vi "NHRDCPower-bak.vi"() -> ()   [LabVIEW 2018, in "Visualization.lvlib" / "VisualizeAcPwr.lvclass"]
doc: "This VI listens for any measurement data associated with the provided PluginName and displays it to the user for analysis. The display is only suitable for data coming from the RoomAlert Plugin."
uses:
  VisualizeAcPwr.lvclass
  VisualizeBase/VisualizeBase_class/SubVIs/VisualizationOptions.ctl
  <vilib>/Utility/miscctls.llb/LVRectTypeDef.ctl
  AcPwr/AcPwrShared/clMeasurmentData.ctl
  <vilib>/event_ctls.llb/usereventprio.ctl
  VisualizeBase/VisualizeBase_class/Requests/VisUserEventType.ctl
  <extravilib>/ChannelInstances/Tag-bool/Write With Abort.vi
  <extravilib>/ChannelInstances/Tag-bool/Read With Abort.vi
  <extravilib>/ChannelInstances/Tag-bool/Instantiate.vi
  <extravilib>/ChannelInstances/Tag-bool/EndpointRead.vi
  <vilib>/Utility/error.llb/Error Cluster From Error Code.vi
  <extravilib>/ChannelInstances/Tag-bool/Endpoint.vi
  <vilib>/ErrorRing/Error Ring.xnode
  <userlib>/NIST/NISTErrorLib/NISTErrorLib.lvlib
  VisualizeBase/VisualizeBase_class/VisualizeBase.lvclass
  <extravilib>/ChannelInstances/Tag-bool.lvlib
  TestClass/Test.lvclass
  Sensor/VisualizeSensor.lvclass
  StatusAndLog/VisualizeStatus.lvclass
  AcPwr/AcPwrShared/AcPwrShared.lvlib
  AcPwr/AcPwrPlugins/ChromaPowerSupplyClass/TypeDefs/Measurements.ctl
  AcPwr/AcPwrPlugins/ChromaPowerSupplyClass/ChromaPowerSupply.lvclass
  AcPwr/AcPwrPlugins/ChromaPowerSupplyClass/TypeDefs/Device(s)Settings.ctl
  AcPwr/AcPwrModule/AcPwrModule.lvlib
  AcPwr/AcPwrPlugins/AcPwrPlugins.lvlib
panel:
  in  "Display":enum16{"Raw Data", "Voltage Vs Current"}(ring)
  in  "btnPause":bool
  out "VisualizationProperties":T1={"PauseAtStartup"=TRUE, "LogData"=FALSE, "LaunchInSubPanel"=TRUE, "FPMonitor"=0, "FPWindowBounds"={"Left"=0, "Top"=0, "Right"=0, "Bottom"=0}, "MonitorBounds"={"Left"=0, "Top"=0, "Right"=0, "Bottom"=0}, "MeasIndices"=[]}
  in  "INIFilePath":path
  in  "ModuleID":i32
  in  "Log Data":bool=TRUE
  in  "btnStop":bool
  in  "btnReset":bool
  in  "btnClearTest":bool
  in  "btnStopModule":bool
  out "XY Graph":cluster{dbl[], dbl[]}(graph)
  out "Chart":waveform(dbl)[](graph)=[{"t0"=timestamp(3657200531.6397257 s since 1904-01-01), "dt"=1.0, "Y"=[46.19]}, {"t0"=timestamp(3657200531.6397257 s since 1904-01-01), "dt"=1.0, "Y"=[2.0]}, {"t0"=timestamp(3657200531.6397257 s since 1904-01-01), "dt"=1.0, "Y"=[60.0]}]
  in  "Current":bool
  in  "Voltage":bool
  in  "Current (A)":dbl
  in  "Voltage (V)":dbl
  out "ErrorArray":errorcluster[](array[cluster])
  out "Incorrect DataType?":bool
  out "String Results":string
  in  "PluginName":string="Sensor.RoomAlert1"
  # "Set Parameter"
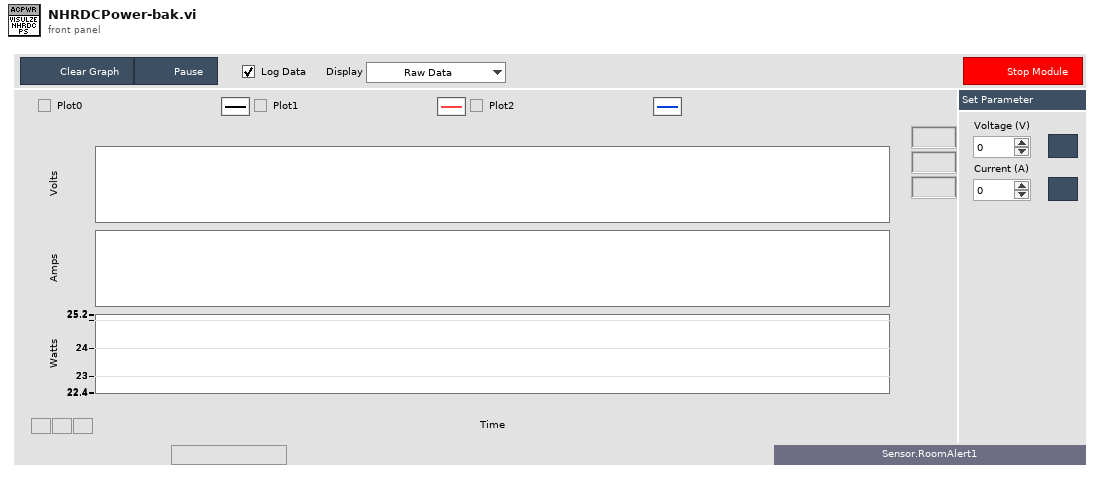
[diagram p1: front panel]
types:
  T1 = typedef "Visualization.lvlib/VisualizeBase.lvclass/VisualizationOptions.ctl" = cluster{"PauseAtStartup":bool, "LogData":bool, "LaunchInSubPanel":bool, "FPMonitor":u16, "FPWindowBounds":T2, "MonitorBounds":cluster{"Left":i16, "Top":i16, "Right":i16, "Bottom":i16}, "MeasIndices":i32[]}
  T2 = typedef "LVRectTypeDef.ctl" = cluster{"Left":i16, "Top":i16, "Right":i16, "Bottom":i16}
  T3 = enum16{"open", "open or create", "create or replace", "create", "open (read-only)"}
  T4 = typedef "Visualization.lvlib/VisualizeBase.lvclass/VisRequestEvents.ctl" = cluster{"StopRequest":refnum<user-event>, "ResetRequest":refnum<user-event>, "FP Pop In or Out":refnum<user-event>}
  T5 = typedef "AcPwrShared.lvlib/AcPwrBroadcastEvents.ctl" = cluster{"DidInit":refnum<user-event>, "StatusUpdate":refnum<user-event>, "ErrorReport":refnum<user-event>, "DidStop":refnum<user-event>, "PathToINI":refnum<user-event>, "Measurements":refnum<user-event>, "LoadConfigFile":refnum<user-event>, "GetSettings":refnum<user-event>, "SetSettings":refnum<user-event>, "GetType&ID":refnum<user-event>, "GotSettings":refnum<user-event>, "GotSettingsLV":refnum<user-event>, "ParameterSet":refnum<user-event>}
  T6 = typedef "Visualization.lvlib/VisualizeBase.lvclass/VisFrmWrkBroadcastEvents.ctl" = cluster{"StatusUpdate":refnum<user-event>, "DidStop":refnum<user-event>, "NewModuleLoaded":refnum<user-event>, "StopVisualization":refnum<user-event>}
  T7 = typedef "AcPwrShared.lvlib/clMeasurmentData.ctl" = cluster{"MeasName":string, "XML Data":string, "WaveformData":waveform(dbl)[]}
  T8 = typedef "AcPwrPlugins.lvlib/ChromaPowerSupply.lvclass/Device(s)Settings.ctl" = cluster{"Phases":cluster{"Handle":string, "Instrument Options":string, "id query (T)":bool, "reset device (T)":bool, "Timing":cluster{"TimingOn":enum16{""}, "Hours":u32, "Minutes":u32, "Seconds":dbl, "CutoffVoltage":dbl}, "Connected":bool, "Output Mode":enum16{"Voltage (DC)", "Current (DC)"}, "Voltage":dbl, "Current":dbl, "High Voltage Limit":dbl, "High Current Limit":dbl, "Power Protect":dbl, "Current Protect":dbl, "Voltage Protect":dbl, "Low Current Limit":dbl, "Low Voltage Limit":dbl, "Current Slew Rate":dbl, "Voltage Slew Rate":dbl, "Current Slew Infinite?":bool}[], "MeasName":string}
  T9 = typedef "AcPwrPlugins.lvlib/ChromaPowerSupply.lvclass/Measurements.ctl" = cluster{"Handle":string, "Name":string, "Enabled":bool, "Measurement Value":dbl, "btnMeasFetch":bool, "ProtectionStatusString":string, "Measurement Type":enum16{"Voltage", "Current", "Power"}}[]
  T10 = typedef "Visualization.lvlib/VisualizeBase.lvclass/VisUserEventType.ctl" = cluster{"BusIndex":i8, "Data":variant}
  T11 = typedef "usereventprio.ctl" = enum32{"high priority", "normal priority"}
  T12 = cluster{"Handle":string, "Instrument Options":string, "id query (T)":bool, "reset device (T)":bool, "Timing":cluster{"TimingOn":enum16{""}, "Hours":u32, "Minutes":u32, "Seconds":dbl, "CutoffVoltage":dbl}, "Connected":bool, "Output Mode":enum16{"Voltage (DC)", "Current (DC)"}, "Voltage":dbl, "Current":dbl, "High Voltage Limit":dbl, "High Current Limit":dbl, "Power Protect":dbl, "Current Protect":dbl, "Voltage Protect":dbl, "Low Current Limit":dbl, "Low Voltage Limit":dbl, "Current Slew Rate":dbl, "Voltage Slew Rate":dbl, "Current Slew Infinite?":bool}[]
  T13 = cluster{"Handle":string, "Instrument Options":string, "id query (T)":bool, "reset device (T)":bool, "Timing":cluster{"TimingOn":enum16{""}, "Hours":u32, "Minutes":u32, "Seconds":dbl, "CutoffVoltage":dbl}, "Connected":bool, "Output Mode":enum16{"Voltage (DC)", "Current (DC)"}, "Voltage":dbl, "Current":dbl, "High Voltage Limit":dbl, "High Current Limit":dbl, "Power Protect":dbl, "Current Protect":dbl, "Voltage Protect":dbl, "Low Current Limit":dbl, "Low Voltage Limit":dbl, "Current Slew Rate":dbl, "Voltage Slew Rate":dbl, "Current Slew Infinite?":bool}
  T14 = typedef "Tag-bool.lvlib/))Channel.ctl" = refnum<queue>
  T15 = typedef "sizeaction.ctl" = enum32{"Minimized", "Maximized", "Resized"}
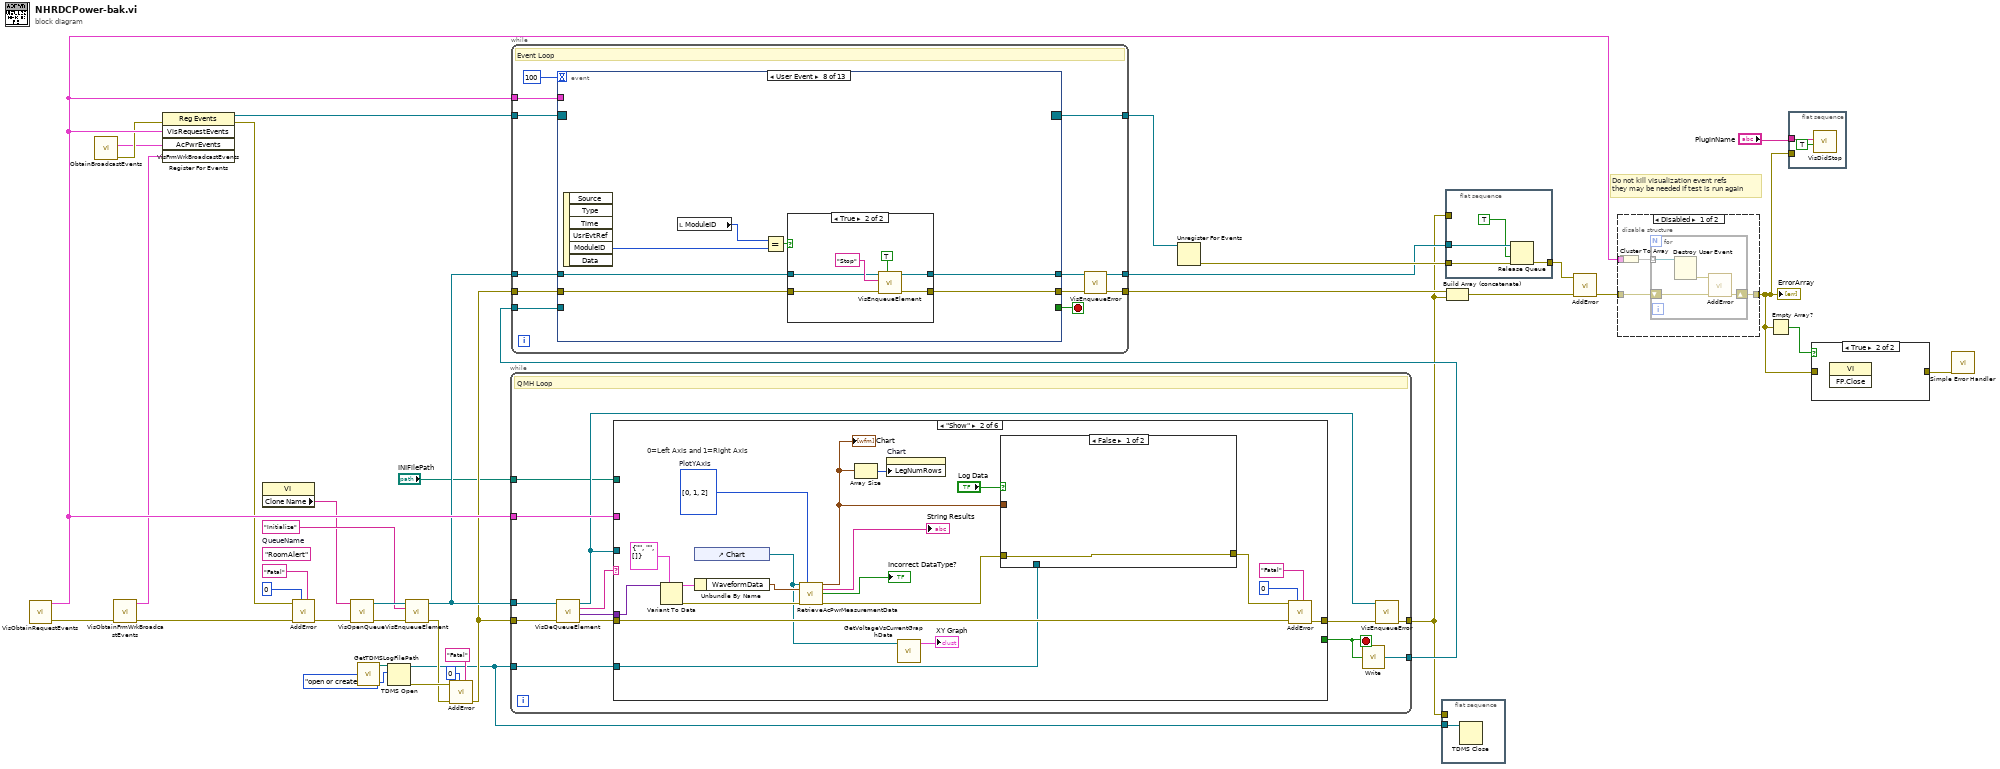
[diagram p0: block diagram]
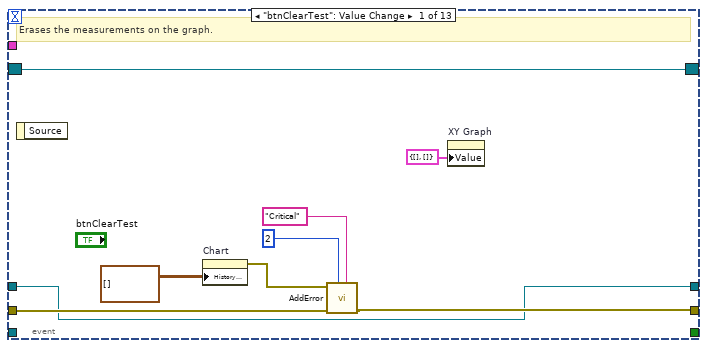
[diagram p3: hidden frame]
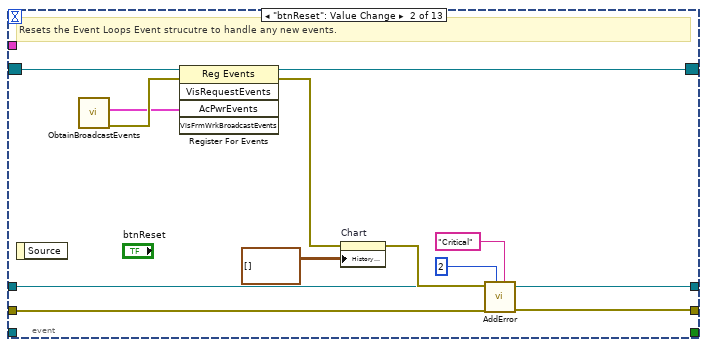
[diagram p4: hidden frame]
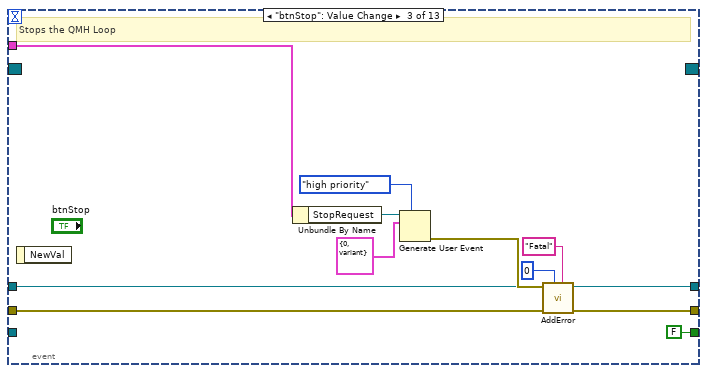
[diagram p5: hidden frame]
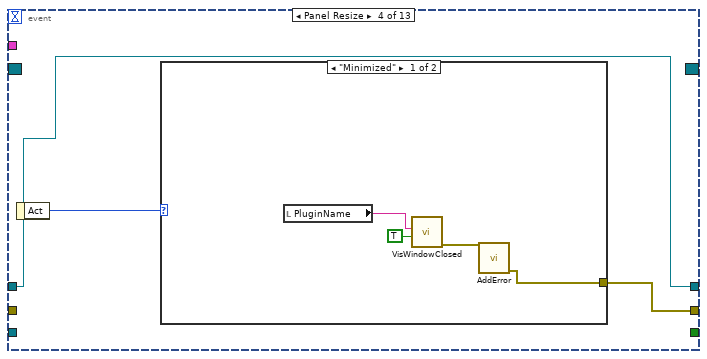
[diagram p6: hidden frame]
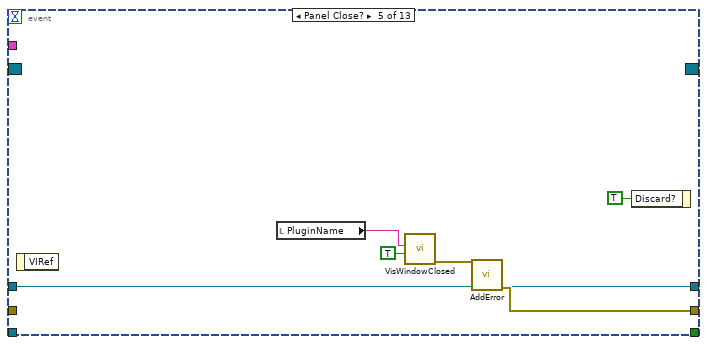
[diagram p8: hidden frame]
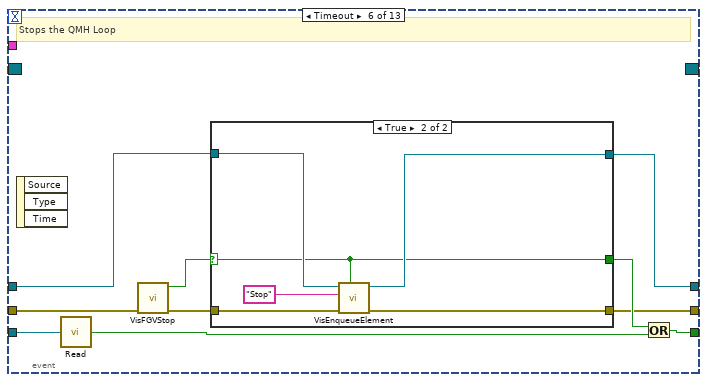
[diagram p9: hidden frame]
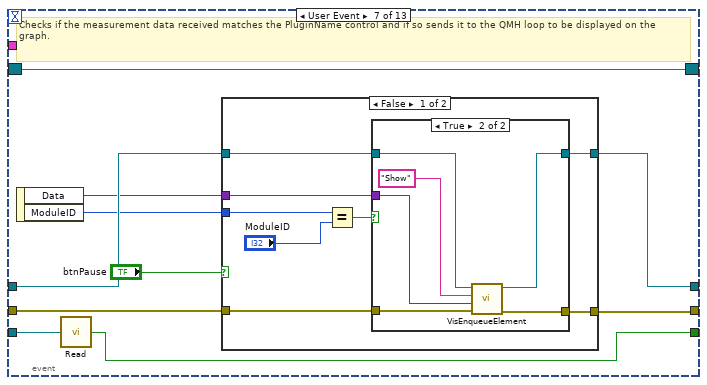
[diagram p11: hidden frame]
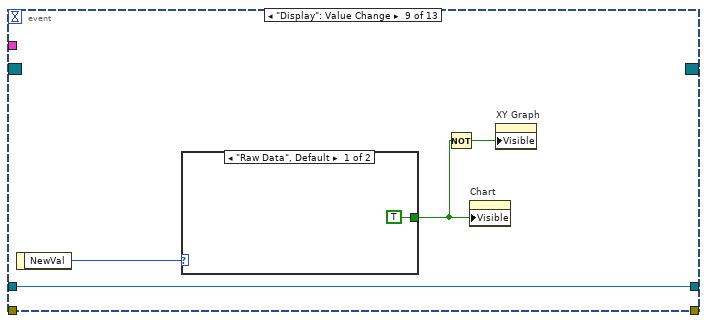
[diagram p15: hidden frame]
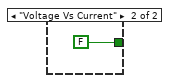
[diagram p16: hidden frame]
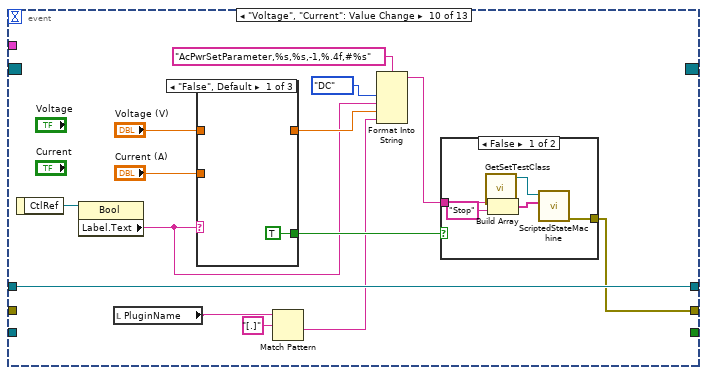
[diagram p17: hidden frame]
diagram:
  (unwired) "RoomAlert"  # QueueName
  # "Do not kill visualization event refs\nthey may be needed if test is run again"
  n1 = call "VisObtainRequestEvents.vi"() -> ("Error"=w29:errorcluster[], "VisRequestEvents"=w31:T4)  [unwired: 10 in]
  n2 = call "ObtainBroadcastEvents.vi"() -> ("error out"=w25:errorcluster, "AcPwrEvents"=w17:T5)  [unwired: 10 in]
  n3 = call "VisObtainFrmWrkBroadcastEvents.vi"("Error"=w29) -> ("Error"=w2:errorcluster[], "VisFrmWrkBroadcastEvents"=w1:T6)  [unwired: 9 in]
  n4 = register-events(error in=w25, w31, w17, w1) -> (reference out=w38:refnum<event-registration>, error out=w28:errorcluster)  [unwired: 1 in]
  n5 = property class="VI"() -> ("Clone Name"=w15:string)  [unwired: 2 in, 2 out]
  n6 = call <userlib>:"AddError.vi"("Severity"="Fatal", "Priority"=u8 0, "ErrorArray In"=w2, "error in (no error)"=w28) -> ("ErrorArray Out"=w24:errorcluster[])  [unwired: 6 in, 1 out]
  n7 = call "VisOpenQueue.vi"("Error Array In"=w24, "QueueName"=w15) -> ("Error Array Out"=w22:errorcluster[], "queue out"=w23:refnum<queue>)  [unwired: 8 in]
  n8 = call "GetTDMSLogFilePath.vi"() -> ("TDMS Log File Path"=w14:path)  [unwired: 11 in]
  n9 = TDMS Open(10:T3."open or create" ("operation (0:open)"), 11:w14) -> (0:w11:errorcluster, 3:w7:refnum<k34>)  [unwired: 5 in]
  n10 = call "VisEnqueueElement.vi"("Error Array In"=w22, "Message"="Initialize", "queue in"=w23) -> ("Error Array Out"=w10:errorcluster[], "queue out"=w20:refnum<queue>)  [unwired: 7 in]
  n11 = call <userlib>:"AddError.vi"("Severity"="Fatal", "Priority"=u8 0, "ErrorArray In"=w10, "error in (no error)"=w11) -> ("ErrorArray Out"=w9:errorcluster[])  [unwired: 6 in, 1 out]
  n12 = while {
    tunnel: w9 -> [w45]
    tunnel: [w48] -> w6
    tunnel: w20 -> [w44]
    tunnel: w31 -> [w50]
    tunnel: [w41] -> w16
    tunnel: w7 -> [w40]
    tunnel: "INIFilePath" -> [w39]
    stop <- w51 stop-if-true
    # "QMH Loop"
    n13 = call "VisDeQueueElement.vi"("Error Array In"=w45, "Queue In"=w44) -> ("Error Array Out"=w43:errorcluster[], "Data"=w46:variant, "Message"=w47:string, "Queue Out"=w42:refnum<queue>)  [unwired: 6 in]
    n14 = case shown="\"Error\"" w47 {
      selector: w47 -> [_ _ _ w122 _ _]
      tunnel: w46 -> [_ w81 w103 _ w141 _]
      tunnel: w43 -> [w62 w84 w102 w120 _ w170]
      tunnel: [w55 w85 w101 w119 w131 w169] -> w49
      tunnel: [_ _ _ _ w137 TRUE] -> w51
      tunnel: w50 -> [_ _ _ _ w136 _]
      tunnel: w42 -> [_ _ _ _ w135 _]
      tunnel: w40 -> [_ w74 _ _ _ _]
      tunnel: w39 -> [w61 _ _ _ _ w171]
      frame "Initialize" {
        n15 = property on="Chart" class="WFChart (strict)"("History Data"=waveform(dbl)[][] []) -> ()  [unwired: 2 in, 2 out]
        n16 = property on="XY Graph" class="XYGraph (strict)"("Value"=cluster{dbl[], dbl[]} {[], []} ("XY Graph")) -> ()  [unwired: 2 in, 2 out]
        n17 = call "ApplyVisOptions.vi"("INIFilePath"=w61) -> ("error out"=w65:errorcluster, "VisualizationProperties"=→"VisualizationProperties":T1)  [unwired: 9 in]
        n18 = call <userlib>:"AddError.vi"("Severity"="Inform", "ErrorArray In"=w62, "error in (no error)"=w65) -> ("ErrorArray Out"=w63:errorcluster[])  [unwired: 7 in, 1 out]
        n19 = property on="Display" class="Enum (strict)"("Val(Sgnl)"="Display") -> ()  [unwired: 2 in, 2 out]
        n20 = local read "ModuleID"() -> (w52:i32)
        n21 = call "GetSettingsRequestLV.vi"("SettingsToGet"=variant, "ModuleID"=w52) -> ("Error Out"=w54:errorcluster)  [unwired: 9 in]
        n22 = call <userlib>:"AddError.vi"("Severity"="Inform", "ErrorArray In"=w63, "error in (no error)"=w54) -> ("ErrorArray Out"=w55:errorcluster[])  [unwired: 7 in, 1 out]
      }
      frame "Show" {
        w78 = u32[] [0, 1, 2]  # PlotYAxis
        # "0=Left Axis and 1=Right Axis"
        n23 = Variant To Data(type=T7 {"MeasName"="", "XML Data"="", "WaveformData"=[]} ("MeasurmentDataCluster"), Variant=w81) -> (data=w79:T7, error out=w80:errorcluster)  [unwired: 1 in]
        n24 = control-ref of="Chart"() -> (w67:refnum<vi>)
        n25 = Unbundle By Name(w79) -> ("WaveformData"=w68:waveform(dbl)[])
        n26 = call "RetrieveAcPwrMeasurementData.vi"("WaveformChartReference"=w67, "PlotYScale"=w78, "WaveformArrayIn"=w68, "error in (no error)"=w80) -> ("WaveformArrayOut"=w70:waveform(dbl)[], "OutputString(Chroma)"=→"String Results":string, "Incorrect DataType?"=→"Incorrect DataType?":bool, "error out"=w77:errorcluster)  [unwired: 7 in, 1 out]
        "Chart" <- w70
        n27 = Array Size(array=w70) -> (size(s)=w71:i32)
        n28 = property on="Chart" class="WFChart (strict)"("LegNumRows"=w71) -> ()  [unwired: 2 in, 2 out]
        n29 = call "GetVoltageVsCurrentGraphData.vi"("WaveformChart in"=w67) -> ("Cluster"=→"XY Graph":cluster{dbl[], dbl[]})  [unwired: 9 in, 1 out]
        n30 = case shown="False" "Log Data" {
          tunnel: w77 -> [w86 w99]
          tunnel: [w86 w100] -> w76
          tunnel: w70 -> [_ w98]
          tunnel: w74 -> [_ w93]
          frame False {
          }
          frame True {
            n31 = call "PrepareWaveformDataForTDMS.vi"("error in (no error)"=w99, "WaveformArray in"=w98) -> ("error out"=w97:errorcluster, "Measurement Data"=w95:dbl[][], "Channel Names"=w96:string[], "TimeStamp"=w88:timestamp)  [unwired: 6 in]
            n32 = local read "PluginName"() -> (w91:string)
            n33 = Build Array(w88) -> (w87:timestamp[])
            n34 = TDMS Write(0:w93, 5:w91, 7:"TimeStamp" ("PluginName"), 9:w87, 11:w97) -> (4:w92:refnum<k34>, 6:w90:string, 15:w94:errorcluster)  [unwired: 1 in, 1 out]
            n35 = TDMS Write(0:w92, 5:w90, 7:w96, 9:w95, 11:w94) -> (15:w100:errorcluster)  [unwired: 1 in, 3 out]
          }
        }
        n36 = call <userlib>:"AddError.vi"("Severity"="Fatal" ("String"), "Priority"=u8 0, "ErrorArray In"=w84, "error in (no error)"=w76) -> ("ErrorArray Out"=w85:errorcluster[])  [unwired: 6 in, 1 out]
      }
      frame "GotSettings" {
        n37 = disable-structure shown="Disabled" {
          disable-tunnel: w103 -> [w111 _]
          disable-tunnel: w102 -> [w109 w115]
          disable-tunnel: [w108 w115] -> w101
          frame Disabled {
            n38 = Variant To Data(type=cluster{"Device Settings":T8, "Measurements":T9} {"Device Settings"={"Phases"=[], "MeasName"=""}, "Measurements"=[]} ("output cluster"), Variant=w111) -> (data=w112:cluster{"Device Settings":T8, "Measurements":T9}, error out=w107:errorcluster)  [unwired: 1 in]
            n39 = Unbundle By Name(w112) -> ("Device Settings.Phases"=w113:T12)
            n40 = Index Array(array=w113) -> (element=w114:T13)  [unwired: 1 in]
            n41 = Unbundle By Name(w114) -> ("Voltage"=w105:dbl, "Current"=w104:dbl)
            n42 = call <userlib>:"AddError.vi"("Severity"="Inform", "ErrorArray In"=w109, "error in (no error)"=w107) -> ("ErrorArray Out"=w108:errorcluster[])  [unwired: 7 in, 1 out]
            n43 = local write "Voltage (V)"(w105) -> ()
            n44 = local write "Current (A)"(w104) -> ()
          }
          frame Enabled {
          }
        }
      }
      frame Default {
        n45 = xnode "Error Ring"("parameter 0"=w122) -> ("error out"=w121:errorcluster)
        n46 = call <userlib>:"AddError.vi"("Severity"="Inform" ("String"), "Priority"=u8 5, "ErrorArray In"=w120, "error in (no error)"=w121) -> ("ErrorArray Out"=w119:errorcluster[], "error out"=w118:errorcluster)  [unwired: 6 in]
        n47 = call <vilib>:"Clear Errors.vi"("error in (no error)"=w118) -> ()  [unwired: 5 in, 2 out]
      }
      frame "Error" {
        n48 = Variant To Data(type=errorcluster[] [], Variant=w141) -> (data=w139:errorcluster[], error out=w130:errorcluster)  [unwired: 1 in]
        n49 = call <userlib>:"ParseErrors.vi"("ErrorArray"=w139) -> ("ErrorArray"=w138:errorcluster[])  [unwired: 8 in, 2 out]
        n50 = for {
          tunnel: w138 -> [w152] mode=indexing
          tunnel: [w146] -> w132 mode=concatenating
          tunnel: [w144] -> w137
          tunnel: w136 -> [w143]
          tunnel: w135 -> [w142]
          stop <- w144 stop-if-true
          n51 = call <userlib>:"GeneralHandler.vi"("error in (no error)"=w152) -> ("Severity"=w145:string, "Stop"=w149:bool, "Abort"=w150:bool, "Continue"=w151:bool)  [unwired: 6 in, 1 out]
          n52 = Build Array(w151, w150, w149) -> (w148:bool[])
          n53 = Boolean Array To Number(Boolean array=w148) -> (number=w147:u32)
          n54 = case shown="1" w147 {
            tunnel: [_ _ w157 w166] -> w146
            tunnel: w145 -> [_ _ _ w159]
            tunnel: [_ _ _ w161] -> w144
            tunnel: w143 -> [_ _ _ w160]
            tunnel: w142 -> [_ _ w153 _]
            frame 0, Default {
              # "No Dialog"
            }
            frame 1 {
              # "Continue"
            }
            frame 2 {
              # "Abort, Flush Queue"
              n55 = Flush Queue(queue=w153) -> (error out=w156:errorcluster)  [unwired: 1 in, 2 out]
              n56 = call <userlib>:"AddError.vi"("Severity"="Critical" ("String"), "Priority"=u8 1, "error in (no error)"=w156) -> ("ErrorArray Out"=w157:errorcluster[])  [unwired: 7 in, 1 out]
            }
            frame 4 {
              # "Stop"
              n57 = Unbundle By Name(w160) -> ("StopRequest"=w167:refnum<user-event>)
              n58 = Equal?(x=w159, y="Fatal" ("x")) -> (x = y?=w161:bool)
              n59 = Generate User Event(priority (normal)=usereventprio."high priority", user event=w167, event data cluster=T10 {"BusIndex"=0, "Data"=variant} ("event data")) -> (error out=w165:errorcluster)  [unwired: 1 in, 1 out]
              n60 = call <userlib>:"AddError.vi"("error in (no error)"=w165) -> ("ErrorArray Out"=w166:errorcluster[], "error out"=w162:errorcluster)  [unwired: 9 in]
              n61 = call <vilib>:"Clear Errors.vi"("error in (no error)"=w162) -> ()  [unwired: 5 in, 2 out]
            }
          }
        }
        n62 = call <userlib>:"AddError.vi"("Severity"="Critical", "Priority"=u8 2, "ErrorArray In"=w132, "error in (no error)"=w130) -> ("ErrorArray Out"=w131:errorcluster[])  [unwired: 6 in, 1 out]
      }
      frame "Stop" {
        n63 = local read "VisualizationProperties"() -> (w168:T1)
        n64 = call "WriteVisOptionsToINIFile.vi"("Visualization Options"=w168, "INIFilePath"=w171) -> ("error out"=w172:errorcluster)  [unwired: 8 in, 1 out]
        n65 = call <userlib>:"AddError.vi"("Severity"="Inform", "ErrorArray In"=w170, "error in (no error)"=w172) -> ("ErrorArray Out"=w169:errorcluster[])  [unwired: 7 in, 1 out]
      }
    }
    n66 = call <extravilib>:"Write.vi"("element"=w51) -> ("channel"=w41:T14)  [unwired: 1 out]
    n67 = call "VisEnqueueError.vi"("Error Array In"=w49, "Queue in"=w42) -> ("Error Array Out"=w48:errorcluster[])  [unwired: 8 in, 1 out]
  }
  n68 = while {
    tunnel: w38 -> [w186]
    tunnel: [w180] -> w36
    tunnel: [w184] -> w37
    tunnel: w31 -> [w183]
    tunnel: w9 -> [w182]
    tunnel: w20 -> [w181]
    tunnel: [w177] -> w19
    tunnel: w16 -> [w175]
    stop <- w185 stop-if-true
    # "Event Loop"
    n69 = event shown="[11] \"btnStopModule\": Value Change" {
      selector: w186 -> [w189 w207 _ _ _ _ w256 _ _ _ _ _ _]
      dyn-events: [w189 w206 _ _ _ _ w256 _ _ _ _ _ _] -> w184
      timeout: 100 -> [_ _ _ _ _ _ _ _ _ _ _ _ _]
      tunnel: [_ _ FALSE ("Priority? (F)") _ _ w232 w253 _ _ _ _ _ _] -> w185
      tunnel: [w192 w204 w211 w220 w227 w234 w258 w282 _ w300 w328 w339 w349] -> w179
      tunnel: w183 -> [_ _ w210 _ _ _ _ _ _ _ _ _ _]
      tunnel: w182 -> [w193 w205 w218 _ _ w237 w259 w281 _ _ w326 _ w348]
      tunnel: w181 -> [w187 w197 w208 w219 w226 w236 w260 w284 w294 w312 w325 w338 w351]
      tunnel: [w187 w197 w208 w219 w226 w235 w257 w283 w294 w312 w327 w338 w350] -> w178
      tunnel: w175 -> [_ _ _ _ _ w241 w254 _ _ _ _ _ _]
      event "btnClearTest": Value Change {
        # "Erases the measurements on the graph."
        n70 = event-data() -> ()  [unwired: 1 in, 1 out]
        n71 = property on="Chart" class="WFChart (strict)"("History Data"=waveform(dbl)[][] []) -> (error out=w191:errorcluster)  [unwired: 2 in, 1 out]
        n72 = call <userlib>:"AddError.vi"("Severity"="Critical", "Priority"=u8 2, "ErrorArray In"=w193, "error in (no error)"=w191) -> ("ErrorArray Out"=w192:errorcluster[])  [unwired: 6 in, 1 out]
        n73 = property on="XY Graph" class="XYGraph (strict)"("Value"=cluster{dbl[], dbl[]} {[], []} ("XY Graph")) -> ()  [unwired: 2 in, 2 out]
      }
      event "btnReset": Value Change {
        # "Resets the Event Loops Event strucutre to handle any new events."
        n74 = event-data() -> ()  [unwired: 1 in, 1 out]
        n75 = call "ObtainBroadcastEvents.vi"() -> ("error out"=w198:errorcluster, "AcPwrEvents"=w196:T5)  [unwired: 10 in]
        n76 = register-events(reference=w207, error in=w198, w196) -> (reference out=w206:refnum<event-registration>, error out=w200:errorcluster)  [unwired: 2 in]
        n77 = property on="Chart" class="WFChart (strict)"(error in=w200, "History Data"=waveform(dbl)[][] []) -> (error out=w199:errorcluster)  [unwired: 1 in, 1 out]
        n78 = call <userlib>:"AddError.vi"("Severity"="Critical", "Priority"=u8 2, "ErrorArray In"=w205, "error in (no error)"=w199) -> ("ErrorArray Out"=w204:errorcluster[])  [unwired: 6 in, 1 out]
      }
      event "btnStop": Value Change {
        # "Stops the QMH Loop"
        n79 = event-data() -> ()  [unwired: 1 in, 1 out]
        n80 = Unbundle By Name(w210) -> ("StopRequest"=w216:refnum<user-event>)
        n81 = Generate User Event(priority (normal)=usereventprio."high priority", user event=w216, event data cluster=T10 {"BusIndex"=0, "Data"=variant} ("event data")) -> (error out=w217:errorcluster)  [unwired: 1 in, 1 out]
        n82 = call <userlib>:"AddError.vi"("Severity"="Fatal" ("String"), "Priority"=u8 0, "ErrorArray In"=w218, "error in (no error)"=w217) -> ("ErrorArray Out"=w211:errorcluster[])  [unwired: 6 in, 1 out]
      }
      event Panel Resize {
        n83 = event-data() -> ("Act"=w221:T15)  [unwired: 1 in]
        n84 = case shown="\"Minimized\"" w221 {
          tunnel: [w222 _] -> w220
          frame "Minimized" {
            n85 = local read "PluginName"() -> (w224:string)
            n86 = call "VisWindowClosed.vi"("Window Closed?"=TRUE ("Window Minimized or Clozed?"), "Module Name"=w224) -> ("error out"=w225:errorcluster)  [unwired: 9 in]
            n87 = call <userlib>:"AddError.vi"("error in (no error)"=w225) -> ("ErrorArray Out"=w222:errorcluster[])  [unwired: 9 in, 1 out]
          }
          frame "Maximized", Default {
          }
        }
      }
      event Panel Close? {
        n88 = event-data() -> ()  [unwired: 1 in, 1 out]
        n89 = local read "PluginName"() -> (w228:string)
        n90 = call "VisWindowClosed.vi"("Window Closed?"=TRUE ("Window Minimized or Clozed?"), "Module Name"=w228) -> ("error out"=w229:errorcluster)  [unwired: 9 in]
        n91 = call <userlib>:"AddError.vi"("error in (no error)"=w229) -> ("ErrorArray Out"=w227:errorcluster[])  [unwired: 9 in, 1 out]
        n92 = event-data("Discard?"=TRUE) -> ()  [unwired: 1 in, 1 out]
      }
      event Timeout {
        # "Stops the QMH Loop"
        n93 = event-data() -> ()  [unwired: 1 in, 3 out]
        n94 = call <extravilib>:"Read.vi"("channel"=w241) -> ("element"=w233:bool)  [unwired: 1 in, 1 out]
        n95 = call "VisFGVStop.vi"("Error In"=w237) -> ("Error Out"=w239:errorcluster[], "Value"=w240:bool)  [unwired: 9 in]
        n96 = case shown="False" w240 {
          selector: w240 -> [w242 w245]
          tunnel: [w244 w248] -> w234
          tunnel: w239 -> [w244 w249]
          tunnel: w236 -> [w243 w247]
          tunnel: [w243 w246] -> w235
          tunnel: [w242 w245] -> w238
          frame False {
          }
          frame True {
            n97 = call "VisEnqueueElement.vi"("Priority? (F)"=w245, "Error Array In"=w249, "Message"="Stop", "queue in"=w247) -> ("Error Array Out"=w248:errorcluster[], "queue out"=w246:refnum<queue>)  [unwired: 6 in]
          }
        }
        n98 = Or(x=w238, y=w233) -> (x .or. y?=w232:bool)
      }
      event User Event {
        # "Checks if the measurement data received matches the PluginName control and if so sends it to the QMH loop to be displayed on the graph."
        n99 = event-data() -> ("Data"=w255:variant, "ModuleID"=w252:i32)  [unwired: 1 in]
        n100 = call <extravilib>:"Read.vi"("channel"=w254) -> ("element"=w253:bool)  [unwired: 1 in, 1 out]
        n101 = case shown="False" "btnPause" {
          tunnel: w260 -> [w268 w278]
          tunnel: w259 -> [w267 w277]
          tunnel: [w266 w277] -> w258
          tunnel: [w265 w278] -> w257
          tunnel: w255 -> [w264 _]
          tunnel: w252 -> [w261 _]
          frame False {
            n102 = Equal?(x=w261, y="ModuleID") -> (x = y?=w263:bool)
            n103 = case shown="True" w263 {
              tunnel: [w269 w275] -> w266
              tunnel: w268 -> [w270 w274]
              tunnel: w267 -> [w269 w276]
              tunnel: [w270 w272] -> w265
              tunnel: w264 -> [_ w273]
              frame False {
              }
              frame True {
                n104 = call "VisEnqueueElement.vi"("Error Array In"=w276, "Data"=w273, "Message"="Show", "queue in"=w274) -> ("Error Array Out"=w275:errorcluster[], "queue out"=w272:refnum<queue>)  [unwired: 6 in]
              }
            }
          }
          frame True {
          }
        }
      }
      event User Event {
        n105 = event-data() -> ("ModuleID"=w280:i32)  [unwired: 1 in, 5 out]
        n106 = local read "ModuleID"() -> (w279:i32)
        n107 = Equal?(x=w279, y=w280) -> (x = y?=w285:bool)
        n108 = case shown="True" w285 {
          tunnel: [w286 w291] -> w282
          tunnel: [w287 w290] -> w283
          tunnel: w284 -> [w287 w289]
          tunnel: w281 -> [w286 w288]
          frame False {
          }
          frame True {
            n109 = call "VisEnqueueElement.vi"("Priority? (F)"=TRUE, "Error Array In"=w288, "Message"="Stop", "queue in"=w289) -> ("Error Array Out"=w291:errorcluster[], "queue out"=w290:refnum<queue>)  [unwired: 6 in]
          }
        }
      }
      event "Display": Value Change {
        n110 = event-data() -> ("NewVal"=w297:enum16{"Raw Data", "Voltage Vs Current"})  [unwired: 1 in]
        n111 = case shown="\"Raw Data\", Default" w297 {
          tunnel: [TRUE FALSE] -> w296
          frame "Raw Data", Default {
          }
          frame "Voltage Vs Current" {
          }
        }
        n112 = Not(x=w296) -> (.not. x?=w295:bool)
        n113 = property on="Chart" class="WFChart (strict)"("Visible"=w296) -> ()  [unwired: 2 in, 2 out]
        n114 = property on="XY Graph" class="XYGraph (strict)"("Visible"=w295) -> ()  [unwired: 2 in, 2 out]
      }
      event "Voltage", "Current": Value Change {
        n115 = event-data() -> ("CtlRef"=w313:refnum<vi>)  [unwired: 1 in]
        n116 = property class="Bool"(reference=w313) -> ("Label.Text"=w302:string)  [unwired: 1 in, 2 out]
        n117 = local read "PluginName"() -> (w305:string)
        n118 = case shown="\"False\", Default" w302 {
          tunnel: "Voltage (V)" -> [_ w320 _]
          tunnel: "Current (A)" -> [_ _ w321]
          tunnel: [_ w320 w321] -> w303
          tunnel: [TRUE _ _] -> w307
          frame "False", Default {
          }
          frame "Voltage" {
          }
          frame "Current" {
          }
        }
        n119 = Match Pattern(string=w305, regular expression="[.]") -> (after substring=w304:string)  [unwired: 1 in, 3 out]
        n120 = Format Into String(format string="AcPwrSetParameter,%s,%s,-1,%.4f,#%s", enum16{"AC", "DC"}."DC" ("input 1"), w302, w303, w304) -> (resulting string=w309:string)  [unwired: 2 in, 1 out]
        n121 = case shown="False" w307 {
          tunnel: w309 -> [w317 _]
          tunnel: [w315 _] -> w300
          frame False {
            n122 = call "GetSetTestClass.vi"() -> ("Test.lvclass"=w318:refnum<class "Test.lvclass">)  [unwired: 11 in]
            n123 = Build Array(w317, "Stop" ("element")) -> (w316:string[])
            n124 = call "ScriptedStateMachine.vi"("script"=w316, "Test.lvclass 2"=w318) -> ("ErrorArray"=w315:errorcluster[])  [unwired: 7 in, 2 out]
          }
          frame True {
          }
        }
      }
      event User Event {
        n125 = event-data() -> ("ModuleID"=w323:i32, "Data"=w322:variant)  [unwired: 1 in]
        n126 = local read "ModuleID"() -> (w324:i32)
        n127 = Equal?(x=w324, y=w323) -> (x = y?=w329:bool)
        n128 = case shown="True" w329 {
          tunnel: w325 -> [w330 w336]
          tunnel: w326 -> [w331 w335]
          tunnel: [w330 w334] -> w327
          tunnel: [w331 w333] -> w328
          tunnel: w322 -> [_ w332]
          frame False {
          }
          frame True {
            (unwired) TRUE ("Priority? (F)")
            n129 = call "VisEnqueueElement.vi"("Error Array In"=w335, "Data"=w332, "Message"="GotSettings", "queue in"=w336) -> ("Error Array Out"=w333:errorcluster[], "queue out"=w334:refnum<queue>)  [unwired: 6 in]
          }
        }
      }
      event "btnStopModule": Value Change {
        n130 = event-data() -> ()  [unwired: 1 in, 1 out]
        n131 = local read "ModuleID"() -> (w341:i32)
        n132 = call "StatusUpdateByModID.vi"("Status"="User requested module stop", "Accessors:Module ID"=w341) -> ("error out"=w342:errorcluster)  [unwired: 9 in]
        n133 = flat-sequence {
          tunnel: [w344] -> w339
          tunnel: w342 -> [_]
          frame #0 {
            n134 = local read "PluginName"() -> (w343:string)
            n135 = call "GetSetTestClass.vi"() -> ("Test.lvclass"=w345:refnum<class "Test.lvclass">)  [unwired: 11 in]
            n136 = call "StopModByName.vi"("Module Name"=w343, "Test.lvclass"=w345) -> ("ErrorArray Out"=w344:errorcluster[])  [unwired: 4 in, 5 out]
          }
        }
      }
      event User Event {
        # "Framework requested visualization stop"
        n137 = event-data() -> ("Data"=w346:variant)  [unwired: 1 in]
        n138 = local read "PluginName"() -> (w347:string)
        n139 = Variant To Data(type="" ("Message"), Variant=w346) -> (data=w357:string, error out=w355:errorcluster)  [unwired: 1 in]
        n140 = call <userlib>:"AddError.vi"("Severity"="Inform", "Priority"=u8 3, "ErrorArray In"=w348, "error in (no error)"=w355) -> ("ErrorArray Out"=w354:errorcluster[])  [unwired: 6 in, 1 out]
        n141 = Equal?(x=w347, y=w357) -> (x = y?=w356:bool)
        n142 = case shown="True" w356 {
          tunnel: w351 -> [w360 w364]
          tunnel: [w359 w363] -> w349
          tunnel: w354 -> [w359 w362]
          tunnel: [w360 w361] -> w350
          frame False {
          }
          frame True {
            n143 = call "VisEnqueueElement.vi"("Priority? (F)"=TRUE, "Error Array In"=w362, "Message"="Stop", "queue in"=w364) -> ("Error Array Out"=w363:errorcluster[], "queue out"=w361:refnum<queue>)  [unwired: 6 in]
          }
        }
      }
    }
    n144 = call "VisEnqueueError.vi"("Error Array In"=w179, "Queue in"=w178) -> ("Error Array Out"=w180:errorcluster[], "Queue out"=w177:refnum<queue>)  [unwired: 8 in]
  }
  n145 = Unregister For Events(event registration refnum=w37) -> (error out=w35:errorcluster)  [unwired: 1 in]
  n146 = flat-sequence {
    tunnel: w7 -> [w367]
    tunnel: w6 -> [_]
    frame #0 {
      n147 = TDMS Close(11:w367) -> ()  [unwired: 1 in, 2 out]
    }
  }
  n148 = flat-sequence {
    tunnel: w35 -> [w371]
    tunnel: [w370] -> w33
    tunnel: w19 -> [w369]
    tunnel: w6 -> [_]
    frame #0 {
      n149 = Release Queue(queue=w369, force destroy? (F)=TRUE, error in (no error)=w371) -> (error out=w370:errorcluster)  [unwired: 2 out]
    }
  }
  n150 = Build Array (concatenate)(w36, w6) -> (w34:errorcluster[])
  n151 = call <userlib>:"AddError.vi"("ErrorArray In"=w34, "error in (no error)"=w33) -> ("ErrorArray Out"=w32:errorcluster[])  [unwired: 8 in, 1 out]
  n152 = disable-structure shown="Disabled" {
    disable-tunnel: w32 -> [w374 w380]
    disable-tunnel: w31 -> [w373 _]
    disable-tunnel: [w372 w380] -> w3
    frame Disabled {
      n153 = Cluster To Array(cluster=w373) -> (array=w375:refnum<user-event>[])
      n154 = for {
        tunnel: w375 -> [w379] mode=indexing
        shift-right: [w378] -> w372
        shift-left: w374 -> [w377]
        n155 = Destroy User Event(user event=w379) -> (error out=w376:errorcluster)  [unwired: 1 in]
        n156 = call <userlib>:"AddError.vi"("ErrorArray In"=w377, "error in (no error)"=w376) -> ("ErrorArray Out"=w378:errorcluster[])  [unwired: 8 in, 1 out]
      }
    }
    frame Enabled {
    }
  }
  "ErrorArray" <- w3
  n157 = Empty Array?(array=w3) -> (empty?=w30:bool)
  n158 = flat-sequence {
    tunnel: "PluginName" -> [w382]
    tunnel: w3 -> [_]
    frame #0 {
      n159 = call "VisDidStop.vi"("DidStop?"=TRUE, "Module Name"=w382) -> ()  [unwired: 9 in, 1 out]
    }
  }
  n160 = case shown="True" w30 {
    tunnel: [w383 _] -> w18
    tunnel: w3 -> [w384 _]
    frame False {
      n161 = Merge Errors(w384) -> (w383:errorcluster)
    }
    frame True {
      n162 = invoke class="VI" method="FP.Close"() -> ()  [unwired: 3 in, 3 out]
    }
  }
  n163 = call <vilib>:"Simple Error Handler.vi"("error in (no error)"=w18) -> ()  [unwired: 4 in, 5 out]
